vi "Configure Template.vi"(8 "error in":errorcluster, 11 "Module Connection Information":T1[](array[typedef])) -> (0 "error out":errorcluster, 2 "Cancelled?":bool, 3 "state configurations":T3=[{"Name"="No Connections", "Description"="State with no connections", "Value"=-1, "Connection List"=[]}], 5 "Routing Channel Name":string)   [LabVIEW 2020, in "Routing and Faulting System Explorer.lvlib"]
uses:
  Routing and Faulting System Explorer.lvlib
  Shared/Channel States.ctl
  Shared/Routing State.ctl
  Shared/Connection.ctl
  Scripting/Types/Module Information.ctl
  Shared/Routing and Faulting Hardware API/Types/Possible Connections for Endpoint.ctl
  Routing Templates/Routing Channel Templates/JSON Routing Channel Template/JSON Routing Channel Template.lvclass
  C:/Users/mjacobso/Desktop/SCM/Routing-Faulting/Source/Routing and Faulting/Routing Templates/Routing Channel Templates/Abstract Routing Channel Template/Abstract Routing Channel Template.lvclass
  Routing Templates/Routing Channel Templates/Abstract Routing Channel Template/Abstract Routing Channel Template.lvclass/Abstract Routing Channel Template.ctl
  Routing Templates/Routing Channel Templates/JSON Routing Channel Template/JSON Routing Channel Template.lvclass/JSON Routing Channel Template.ctl
  Routing Templates/Routing Channel Templates/Abstract Routing Channel Template/Write Channel Definition.vi
  Routing Templates/Routing Channel Templates/JSON Routing Channel Template/Write Full Module Name.vi
  Routing Templates/Routing Channel Templates/JSON Routing Channel Template/Read Routing Channel Name.vi
  Shared/Routing and Faulting Shared.lvlib
  Shared/Routing and Faulting Hardware API/Routing and Faulting Hardware API.lvlib
  Scripting/Routing and Faulting Scripting.lvlib
panel:
  in  "Channel Definitions":cluster{"Channel":string, "Source":string}[](array[cluster])
  in  "Templates":string(combo)
  in  "Module":string(combo)
  in  "OK Button":bool
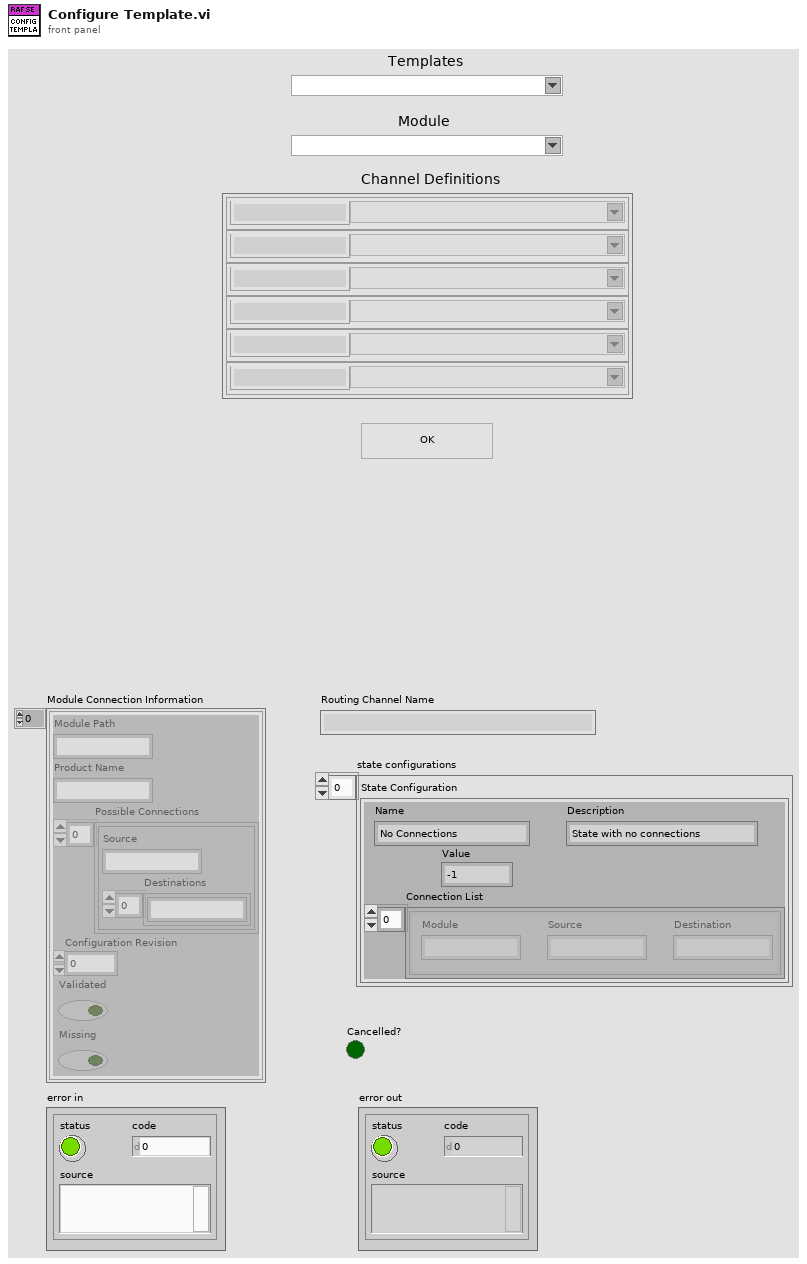
[diagram p1: front panel]
types:
  T1 = typedef "Routing and Faulting Scripting.lvlib/Module Information.ctl" = cluster{"Module Path":string, "Product Name":string, "Possible Connections":T2[], "Configuration Revision":u32, "Validated":bool, "Missing":bool}
  T2 = typedef "Routing and Faulting Hardware API.lvlib/Possible Connections for Endpoint.ctl" = cluster{"Source":string, "Destinations":string[]}
  T3 = typedef "Routing and Faulting Shared.lvlib/Channel States.ctl" = T4[]
  T4 = typedef "Routing and Faulting Shared.lvlib/Routing State.ctl" = cluster{"Name":string, "Description":string, "Value":i32, "Connection List":T5[]}
  T5 = typedef "Routing and Faulting Shared.lvlib/Connection.ctl" = cluster{"Module":string, "Source":string, "Destination":string}
  T6 = cluster{"Module Idx":i32, "JSON Templates":refnum<class "JSON Routing Channel Template.lvclass">[], "Template Idx":i32}
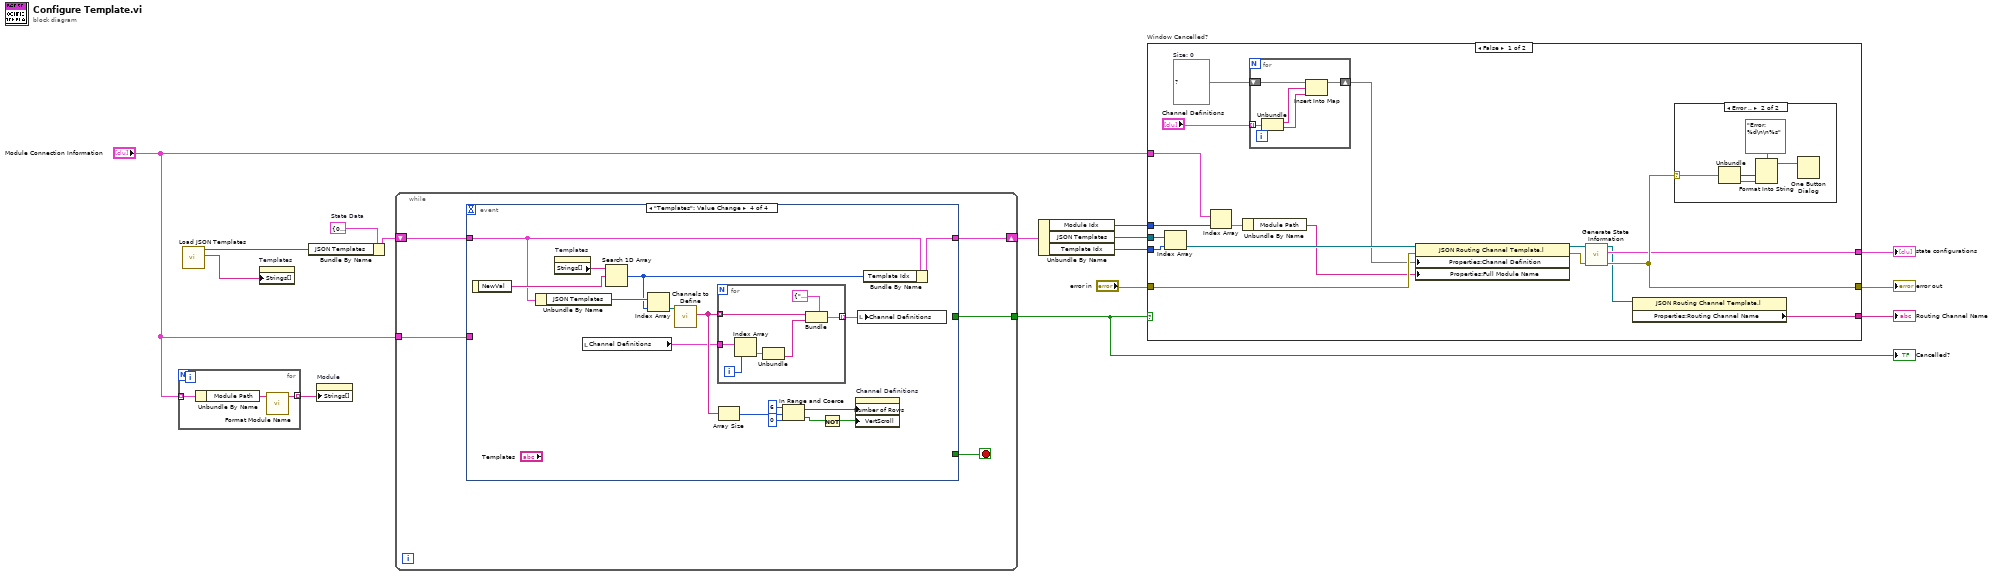
[diagram p0: block diagram]
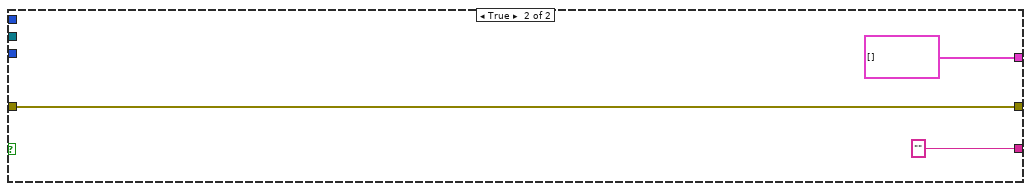
[diagram p3: hidden frame]
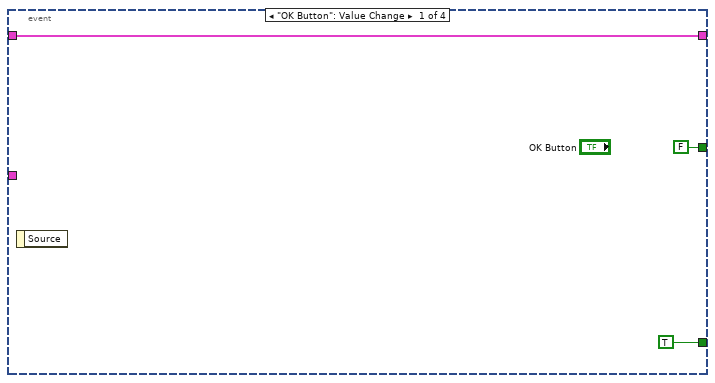
[diagram p4: hidden frame]
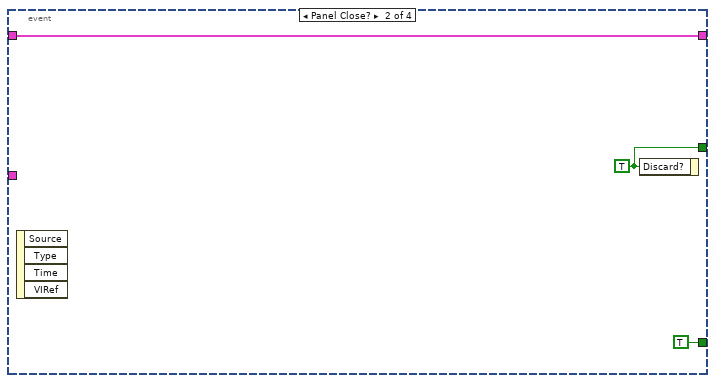
[diagram p5: hidden frame]
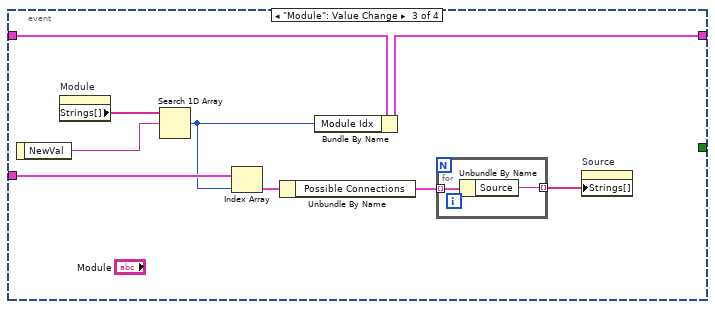
[diagram p6: hidden frame]
diagram:
  w14 = T6 {"Module Idx"=0, "JSON Templates"=[], "Template Idx"=0}  # State Data
  n1 = for {
    tunnel: "Module Connection Information" -> [w18] mode=indexing
    tunnel: [w16] -> w15 mode=indexing
    n2 = Unbundle By Name(w18) -> ("Module Path"=w17:string)
    n3 = call "Format Module Name.vi"("Module Path"=w17) -> ("Formatted Module Path"=w16:string)  [unwired: 10 in]
  }
  n4 = call "Load JSON Templates.vi"() -> ("JSON Template Names"=w9:string[], "JSON Templates"=w8:refnum<class "JSON Routing Channel Template.lvclass">[])  [unwired: 10 in]
  n5 = property on="Templates" class="CmbBox"("Strings[]"=w9) -> ()  [unwired: 2 in, 2 out]
  n6 = Bundle By Name(cluster=w14, "JSON Templates"=w8) -> (w10:T6)
  n7 = property on="Module" class="CmbBox"("Strings[]"=w15) -> ()  [unwired: 2 in, 2 out]
  n8 = while {
    tunnel: [w23] -> w1
    tunnel: "Module Connection Information" -> [w22]
    shift-right: [w19] -> w13
    shift-left: w10 -> [w20]
    stop <- w21 stop-if-true
    n9 = event shown="[3] \"Templates\": Value Change" {
      selector: _ -> [_ _ _ _]
      dyn-events: _ -> [_ _ _ _]
      timeout: _ -> [_ _ _ _]
      tunnel: [FALSE ("Discard?") w29 _ _] -> w23
      tunnel: w22 -> [_ _ w36 _]
      tunnel: [TRUE TRUE _ _] -> w21
      tunnel: w20 -> [w24 w27 w33 w53]
      tunnel: [w24 w27 w32 w54] -> w19
      event "OK Button": Value Change {
        n10 = event-data() -> ()  [unwired: 1 in, 1 out]
      }
      event Panel Close? {
        w29 = TRUE ("Discard?")
        n11 = event-data() -> ()  [unwired: 1 in, 4 out]
        n12 = event-data("Discard?"=w29) -> ()  [unwired: 1 in, 1 out]
      }
      event "Module": Value Change {
        n13 = event-data() -> ("NewVal"=w37:string)  [unwired: 1 in]
        n14 = property on="Module" class="CmbBox"() -> ("Strings[]"=w38:string[])  [unwired: 2 in, 2 out]
        n15 = Search 1D Array(1D array=w38, element=w37) -> (index of element=w31:i32)  [unwired: 1 in]
        n16 = Index Array(array=w36, index=w31) -> (element=w35:T1)
        n17 = Unbundle By Name(w35) -> ("Possible Connections"=w34:T2[])
        n18 = Bundle By Name(cluster=w33, "Module Idx"=w31) -> (w32:T6)
        n19 = for {
          tunnel: w34 -> [w40] mode=indexing
          tunnel: [w39] -> w30 mode=indexing
          n20 = Unbundle By Name(w40) -> ("Source"=w39:string)
        }
        n21 = property on="Source" class="CmbBox"("Strings[]"=w30) -> ()  [unwired: 2 in, 2 out]
      }
      event "Templates": Value Change {
        n22 = event-data() -> ("NewVal"=w55:string)  [unwired: 1 in]
        n23 = Unbundle By Name(w53) -> ("JSON Templates"=w52:refnum<class "JSON Routing Channel Template.lvclass">[])
        n24 = property on="Templates" class="CmbBox"() -> ("Strings[]"=w56:string[])  [unwired: 2 in, 2 out]
        n25 = local read "Channel Definitions"() -> (w48:cluster{"Channel":string, "Source":string}[])
        n26 = Search 1D Array(1D array=w56, element=w55) -> (index of element=w51:i32)  [unwired: 1 in]
        n27 = Index Array(array=w52, index=w51) -> (element=w50:refnum<class "JSON Routing Channel Template.lvclass">)
        n28 = call-dynamic "Channels to Define.vi"("JSON Routing Channel Template in"=w50) -> ("Channels"=w49:string[])  [unwired: 8 in, 2 out]
        n29 = for {
          tunnel: w49 -> [w62] mode=indexing
          tunnel: w48 -> [w59]
          tunnel: [w60] -> w47 mode=indexing
          i -> [w57]
          n30 = Index Array(array=w59, index=w57) -> (element=w58:cluster{"Channel":string, "Source":string})
          n31 = Unbundle(w58) -> ("Source"=w61:string)  [unwired: 1 out]
          n32 = Bundle(cluster=cluster{"Channel":string, "Source":string} {"Channel"="", "Source"=""} ("Channel Definition"), "Channel"=w62, "Source"=w61) -> (w60:cluster{"Channel":string, "Source":string})
        }
        n33 = Array Size(array=w49) -> (size(s)=w46:i32)
        n34 = In Range and Coerce(upper limit=6, x=w46, lower limit=0) -> (coerced(x)=w43:i32, In Range?=w42:bool)
        n35 = Not(x=w42) -> (.not. x?=w41:bool)
        n36 = property on="Channel Definitions" class="Arr (strict)"("Number of Rows"=w43, "VertScroll"=w41) -> ()  [unwired: 2 in, 2 out]
        n37 = local write "Channel Definitions"(w47) -> ()
        n38 = Bundle By Name(cluster=w53, "Template Idx"=w51) -> (w54:T6)
      }
    }
  }
  "Cancelled?" <- w1
  n39 = Unbundle By Name(w13) -> ("Module Idx"=w12:i32, "JSON Templates"=w7:refnum<class "JSON Routing Channel Template.lvclass">[], "Template Idx"=w6:i32)
  n40 = case "Window Cancelled?" shown="False" w1 {
    tunnel: w12 -> [w80 _]
    tunnel: "Module Connection Information" -> [w79 _]
    tunnel: w7 -> [w78 _]
    tunnel: w6 -> [w77 _]
    tunnel: [w76 "" ("Properties:Routing Channel Name")] -> w5
    tunnel: [w75 w93] -> w4
    tunnel: [w74 T4[] [] ("State Configurations")] -> w3
    tunnel: "error in" -> [w73 w93]
    frame False {
      w66 = map{string, string} {}  # Size: 0
      n41 = Index Array(array=w78, index=w77) -> (element=w71:refnum<class "JSON Routing Channel Template.lvclass">)
      n42 = Index Array(array=w79, index=w80) -> (element=w68:T1)
      n43 = Unbundle By Name(w68) -> ("Module Path"=w67:string)
      n44 = for {
        tunnel: "Channel Definitions" -> [w89] mode=indexing
        shift-right: [w86] -> w65
        shift-left: w66 -> [w90]
        n45 = Unbundle(w89) -> ("Channel"=w88:string, "Source"=w87:string)
        n46 = Insert Into Map(map in=w90, key=w88, value=w87) -> (map out=w86:map{string, string})  [unwired: 2 out]
      }
      n47 = property class="JSON Routing Channel Template.l"(reference=w71, error in=w73, "Properties:Channel Definition"=w65, "Properties:Full Module Name"=w67) -> (reference out=w70:refnum<class "JSON Routing Channel Template.lvclass">, error out=w69:errorcluster)
      n48 = call-dynamic "Generate State Information.vi"("error in (no error)"=w69, "JSON RCT"=w70) -> ("error out"=w75:errorcluster, "State Configurations"=w74:T4[], "JSON RCT"=w64:refnum<class "JSON Routing Channel Template.lvclass">)  [unwired: 7 in]
      n49 = property class="JSON Routing Channel Template.l"(reference=w64) -> ("Properties:Routing Channel Name"=w76:string)  [unwired: 1 in, 2 out]
      n50 = case shown="Error .." w75 {
        selector: w75 -> [_ w85]
        frame No Error {
        }
        frame Error {
          n51 = Unbundle(w85) -> ("code"=w83:i32, "source"=w82:string)  [unwired: 1 out]
          n52 = Format Into String(format string="Error: %d\n\n%s", w83, w82) -> (resulting string=w81:string)  [unwired: 2 in, 1 out]
          n53 = One Button Dialog(message=w81) -> ()  [unwired: 1 in, 1 out]
        }
      }
    }
    frame True {
    }
  }
  "state configurations" <- w3
  "error out" <- w4
  "Routing Channel Name" <- w5
